vi "UDcluster Array to String Array.vi"(0 "Array in":T1[](array[typedef]), 11 "error in (no error)":errorcluster) -> (4 "Array out":string[](array[string]), 15 "error out":errorcluster)   [LabVIEW 2012]
uses:
  typedef/User_Data_Cluster.ctl
  typedef/User Accounts.ctl
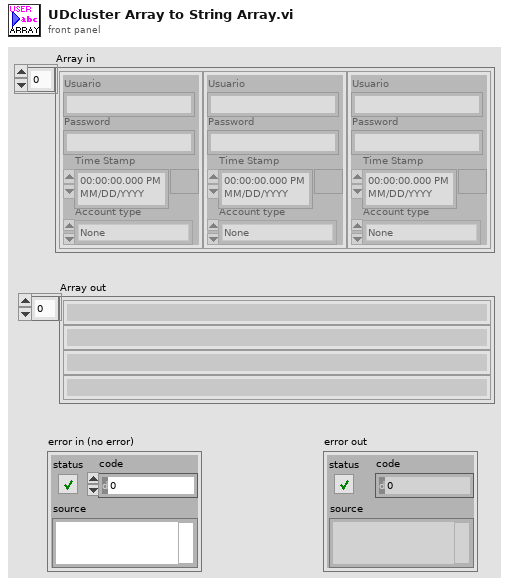
[diagram p1: front panel]
types:
  T1 = typedef "User_Data_Cluster.ctl" = cluster{"Usuario":string, "Password":string, "Account type":T2, "Time Stamp":timestamp}
  T2 = typedef "User Accounts.ctl" = enum16{"None", "User", "Admin"}
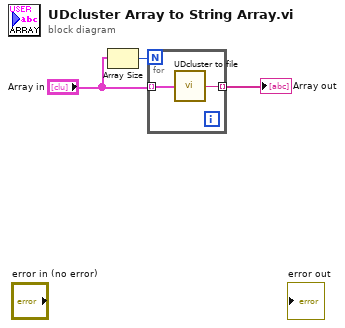
[diagram p0: block diagram]
diagram:
  n1 = Array Size(array="Array in") -> (size(s)=w1:i32)
  n2 = for {
    N: w1 -> [_]
    tunnel: "Array in" -> [w5] mode=indexing
    tunnel: [w4] -> w3 mode=indexing
    n3 = call "UDcluster to file.vi"("User-data cluster"=w5) -> ("CypheredText"=w4:string)
  }
  "Array out" <- w3
